vi "Begin.vi"(8 "error in":errorcluster) -> (0 "error out":errorcluster)   [LabVIEW 2016]
doc: "Called before other user functions, this VI is expected to open initial I/O refnums, load in file data, and do all program initialization. Notice that the <B>error out</B> terminal is simply used for data flow. Wiring it to other structures or subVIs ensures that this VI runs first."
uses:
  <vilib>/Rock Robotics/WPI/SafetyOutput/WPI_SafetyOutputConfigMenu.ctl
  <vilib>/Rock Robotics/WPI/DriverStation/WPI_DriverStationRobotMode2.ctl
  <vilib>/Rock Robotics/WPI/Joystick/WPI_JoystickDeviceEnum.ctl
  <vilib>/Rock Robotics/SystemInterfaces/DIO/FPGA_DIOPWMChannel.ctl
  <vilib>/Rock Robotics/WPI/ThirdParty/CanMotor/TalonSRX/WPI_CANTalonSRX_APIControlMode.ctl
  <vilib>/Rock Robotics/WPI/ThirdParty/CanMotor/TalonSRX/WPI_CANTalonSRX_APIFeedbackSelect.ctl
  navx-mxp/labview/NI WPI/WPI_SerialPort_USB.ctl
  navx-mxp/labview/navX Library v2/TypeDefs/Z900_navX_SerialStreamTypeDef.ctl
  <vilib>/Rock Robotics/SystemInterfaces/DIO/FPGA_DIORelayChannel.ctl
  <vilib>/Rock Robotics/SystemInterfaces/DIO/FPGA_DIOChannel.ctl
  <vilib>/Rock Robotics/WPI/Relay/WPI_RelayValue.ctl
  <vilib>/Rock Robotics/WPI/ThirdParty/CanMotor/TalonSRX/WPI_CANTalonSRX_BrakeOverride.ctl
  Robot Global Data.vi
  <vilib>/Rock Robotics/Network Tables/NT Write String Array.vi
  <vilib>/Rock Robotics/WPI/MotorControl/WPI_MotorControlOpen Victor.vi
  navx-mxp/labview/navX Library v2/IO/Open/Z900_navX_Open_Serial.vi
  <vilib>/Rock Robotics/WPI/Switch/WPI_SwitchOpenLimit.vi
  navx-mxp/labview/navX Library v2/navX Library v2.lvlib
  navx-mxp/labview/NI WPI/NI WPI Serial USB.lvlib
  <vilib>/Rock Robotics/SystemInterfaces/i2clib/i2c_bus.ctl
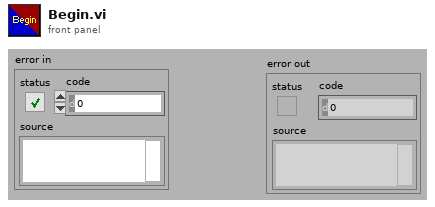
[diagram p1: front panel]
types:
  T1 = typedef "WPI_CANTalonSRX_BrakeOverride.ctl" = enum8{"No Override", "Override to Coast", "Override to Brake"}
  T2 = typedef "WPI_RelayValue.ctl" = enum16{"Off", "On", "Forward", "Reverse"}
  T3 = typedef "FPGA_DIORelayChannel.ctl" = enum8{"Relay 0", "Relay 1", "Relay 2", "Relay 3", "Invalid"}
  T4 = typedef "WPI_JoystickDeviceEnum.ctl" = enum16{"USB 0", "USB 1", "USB 2", "USB 3", "USB 4", "USB 5"}
  T5 = typedef "FPGA_DIOChannel.ctl" = enum8{"DIO 0", "DIO 1", "DIO 2", "DIO 3", "DIO 4", "DIO 5", "DIO 6", "DIO 7", "DIO 8", "DIO 9", "DIO MXP 0", "DIO MXP 1", "DIO MXP 2", "DIO MXP 3", "DIO MXP 4", "DIO MXP 5", "DIO MXP 6", "DIO MXP 7", "DIO MXP 8", "DIO MXP 9", "DIO MXP 10", "DIO MXP 11", "DIO MXP 12", "DIO MXP 13", "DIO MXP 14", "DIO MXP 15", "SPI Port CS1", "SPI Port CS2", "SPI Port CS3", "SPI Port MISO", "SPI Port MOSI", "Invalid"}
  T6 = typedef "WPI_CANTalonSRX_APIFeedbackSelect.ctl" = enum16{"Digital Quadrature Encoder", "Analog Potentiometer", "Analog Encoder", "Count on Quad-A (Rising-Edge)", "Count on Quad-A (Falling-Edge)", "CTR Magnetic Enc (Absolute)", "CTR Magnetic Enc (Relative)", "Pulse Width"}
  T7 = typedef "WPI_CANTalonSRX_APIControlMode.ctl" = enum8{"Percent VBus", "Speed", "Position", "Slave", "Unchanged / Invalid", "Voltage Compensation", "Current", "Motion Profile", "Motion Magic"}
  T8 = typedef "FPGA_DIOPWMChannel.ctl" = enum8{"PWM 0", "PWM 1", "PWM 2", "PWM 3", "PWM 4", "PWM 5", "PWM 6", "PWM 7", "PWM 8", "PWM 9", "PWM MXP 0", "PWM MXP 1", "PWM MXP 2", "PWM MXP 3", "PWM MXP 4", "PWM MXP 5", "PWM MXP 6", "PWM MXP 7", "PWM MXP 8", "PWM MXP 9", "Invalid"}
  T9 = typedef "navX Library v2.lvlib/Z900_navX_SerialStreamTypeDef.ctl" = enum16{"YRPH", "Quaterinons", "Gyro/Raw", "AHRS", "AHRSAndPositioning"}
  T10 = typedef "NI WPI Serial USB.lvlib/WPI_SerialPort_USB.ctl" = enum16{"Onboard RS-232", "MXP TTL", "USB"}
  T11 = typedef "WPI_DriverStationRobotMode2.ctl" = enum16{"Autonomous Disabled", "Autonomous Enabled", "Teleop Disabled", "Teleop Enabled", "Disconnected", "Finish", "Test Disabled", "Test Enabled", "Emergency Stopped"}
  T12 = typedef "WPI_SafetyOutputConfigMenu.ctl" = enum16{"Enable", "Disable"}
  T13 = typedef "i2c_bus.ctl" = enum16{"I2C On-Board", "I2C MXP", "Invalid"}
  T14 = typedef "WPI_I2CDevRef.ctl" = cluster{"DevStatus":errorcluster, "Device Address":u8, "Handle":i32, "I2C Bus":T13}
  T15 = typedef "WPI_JoystickDevRef.ctl" = cluster{"Device":T4}
  T16 = typedef "WPI_RobotDriveDevRef.ctl" = cluster{"DevStatus":errorcluster, "Motors[]":T17[], "Square Inputs":bool, "Max Output":dbl}
  T17 = typedef "WPI_MotorControlDeviceRef.ctl" = cluster{"DeviceStatus":errorcluster, "Type":T18, "PWM":cluster{"PWM Channel":T8, "DeadBand":T19}, "CAN":cluster{"Device Number":u8, "SetOutput VI Ref":variant, "GetOutput VI Ref":variant, "Enable VI Ref":variant, "Disable VI Ref":variant, "Data":variant}, "Invert":bool}
  T18 = typedef "WPI_MotorControlType.ctl" = enum16{"PWM", "CAN"}
  T19 = typedef "WPI_PWMDeadband.ctl" = cluster{"Name":string, "maxPositivePwm":i32, "minPositivePwm":i32, "centerPwm":i32, "maxNegativePwm":i32, "minNegativePwm":i32, "angularRange":u16}
  T20 = typedef "navX Library v2.lvlib/Z900_navX_DeviceTypeDef.ctl" = cluster{"Interface":cluster{"Protocol":T21, "Update Rate (4Hz-100Hz)":u8, "navX Open TypeDef":variant}, "Notify Packet":refnum<notifier>, "Loop VI Refnum":refnum<vi>, "Ready to Close Occurrence Refnum":refnum<k4>}
  T21 = typedef "navX Library v2.lvlib/Z900_navX_ProtocolTypeDef.ctl" = enum16{"SERIAL", "I2C", "SPI"}
  T22 = typedef "WPI_SwitchDevRef.ctl" = cluster{"DevStatus":errorcluster, "DIO Channel":T5, "CntIndex":T23, "Normally Closed":bool}
  T23 = typedef "FPGA_CounterCtrSystemIndex.ctl" = enum8{"Ctr 0", "Ctr 1", "Ctr 2", "Ctr 3", "Ctr 4", "Ctr 5", "Ctr 6", "Ctr 7", "Invalid"}
  T24 = typedef "WPI_RelayDevRef.ctl" = cluster{"DevStatus":errorcluster, "Relay Channel":T3, "Relay Direction":T25}
  T25 = typedef "WPI_RelayDirection.ctl" = enum16{"Both directions", "Forward only", "Reverse only"}
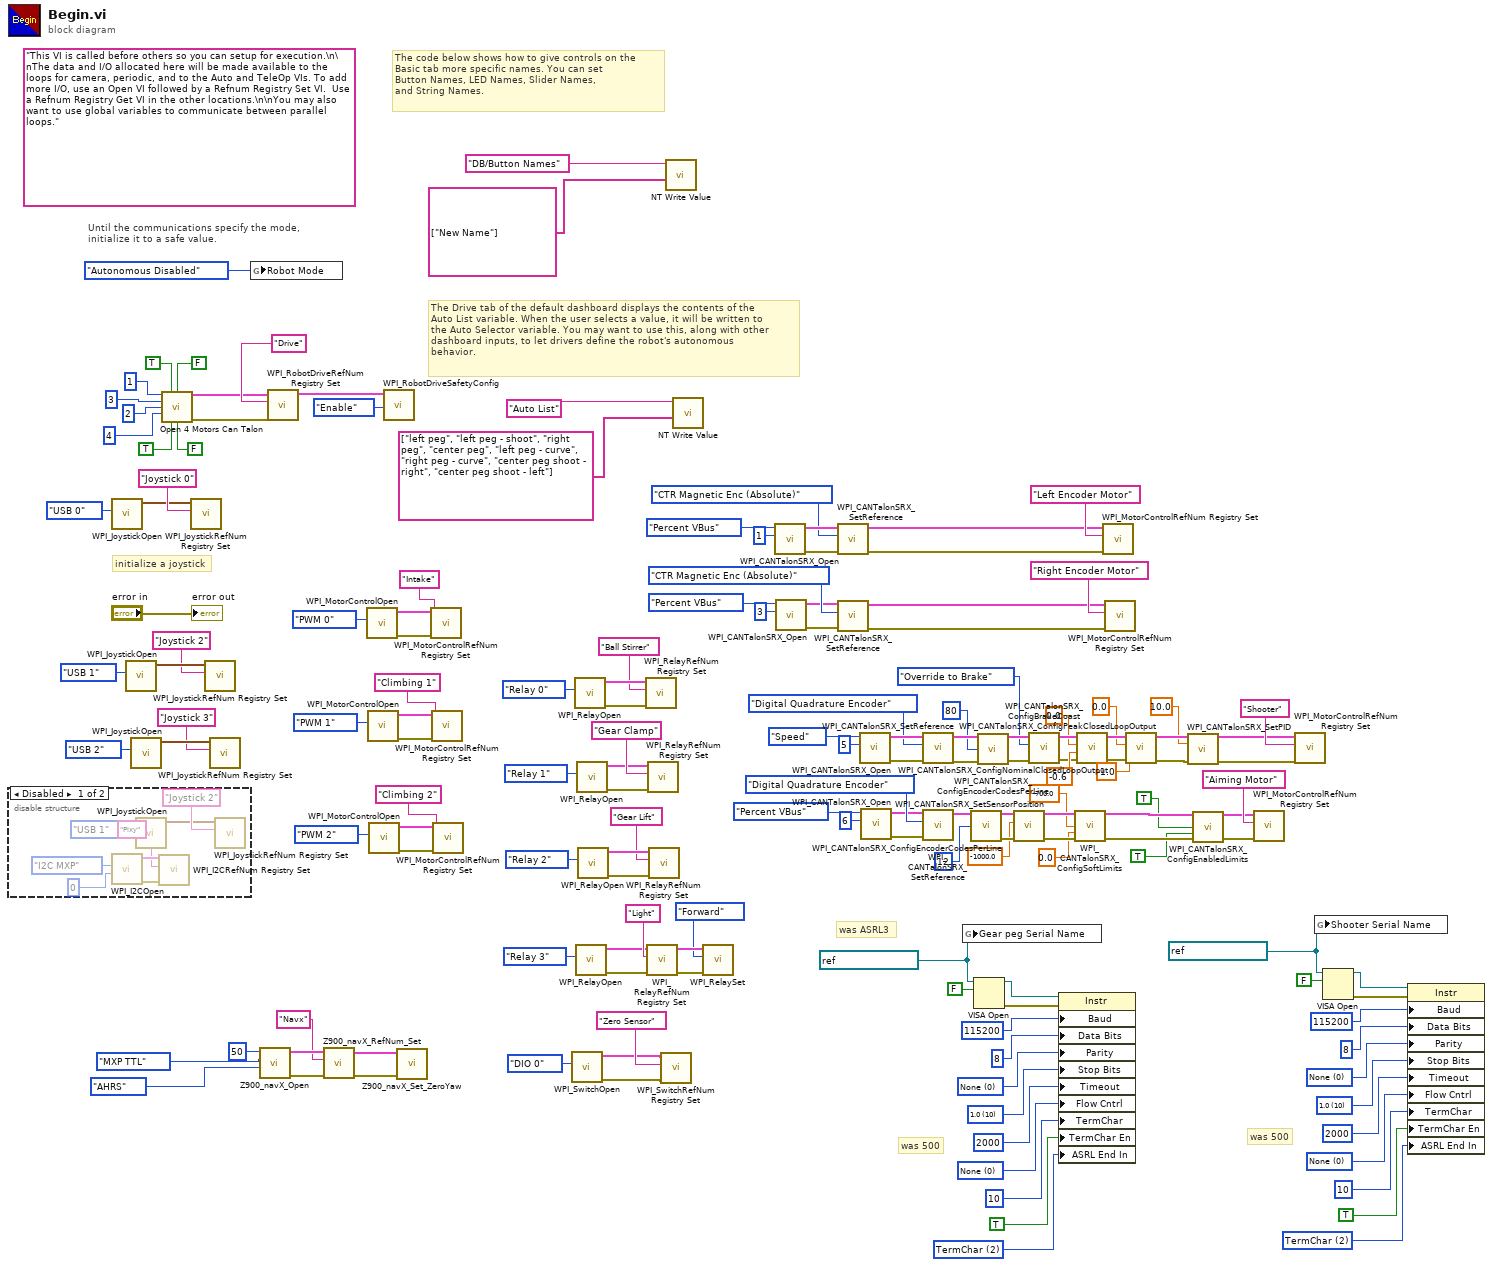
[diagram p0: block diagram]
diagram:
  w30 = refnum<visa-resource-name> "ASRL3::INSTR" ("VISA Refnum out")
  w29 = u16 2 items=["None", "Last Bit", "TermChar"] ("Serial Settings:End Mode for Reads")
  w26 = u16 0 items=["None", "XON/XOFF", "RTS/CTS", "XON/XOFF & RTS/CTS", "DTR/DSR", "XON/XOFF & DTR/DSR"] ("Flow Control")
  w24 = u16 10 items=["1.0"=10, "1.5"=15, "2.0"=20] ("Stop Bits")
  w23 = u16 0 items=["None", "Odd", "Even", "Mark", "Space"] ("Parity")
  w102 = refnum<visa-resource-name> "ASRL4::INSTR" ("VISA Refnum out")
  w103 = u16 2 items=["None", "Last Bit", "TermChar"] ("Serial Settings:End Mode for Reads")
  w106 = u16 0 items=["None", "XON/XOFF", "RTS/CTS", "XON/XOFF & RTS/CTS", "DTR/DSR", "XON/XOFF & DTR/DSR"] ("Flow Control")
  w108 = u16 10 items=["1.0"=10, "1.5"=15, "2.0"=20] ("Stop Bits")
  w109 = u16 0 items=["None", "Odd", "Even", "Mark", "Space"] ("Parity")
  (unwired) "This VI is called before others so you can setup for execution.\n\nThe data and I/O allocated here will be made available to the loops for camera, periodic, and to the Auto and TeleOp VIs. To add more I/O, use an Open VI followed by a Refnum Registry Set VI.  Use a Refnum Registry Get VI in the other locations.\n\nYou may also want to use global variables to communicate between parallel loops."
  # "was ASRL3"
  # "was 500"
  # "was 500"
  # "The Drive tab of the default dashboard displays the contents of the\nAuto List variable. When the user selects a value, it will be written to\nthe Auto Selector variable. You may want to use this, along with other\ndashboard inputs, to let drivers define the robot's autonomous\nbehavior."
  # "The code below shows how to give controls on the\nBasic tab more specific names. You can set\nButton Names, LED Names, Slider Names,\nand String Names."
  # "initialize a joystick"
  # "Until the communications specify the mode,\ninitialize it to a safe value."
  n1 = disable-structure shown="Disabled" {
    frame Disabled {
      n2 = call <vilib>:"WPI_I2COpen.vi"("Device Address"=u8 0, "I2C Bus"=i2c_bus."I2C MXP") -> ("error out"=w162:errorcluster, "I2CDevRef"=w161:T14)  [unwired: 8 in]
      n3 = call <vilib>:"WPI_JoystickOpen.vi"("JoystickDevice"=WPI_JoystickDeviceEnum."USB 1") -> ("JoystickDevRef"=w158:T15)  [unwired: 10 in]
      n4 = call <vilib>:"WPI_I2CRefNum Registry Set.vi"("error in (no error)"=w162, "refnum name"="Pixy", "I2CDevRef"=w161) -> ()  [unwired: 7 in, 2 out]
      n5 = call <vilib>:"WPI_JoystickRefNum Registry Set.vi"("refnum name"="Joystick 2", "JoystickDevRef"=w158) -> ()  [unwired: 8 in, 2 out]
    }
    frame Enabled {
    }
  }
  n6 = call <vilib>:"WPI_JoystickOpen.vi"("JoystickDevice"=WPI_JoystickDeviceEnum."USB 0") -> ("JoystickDevRef"=w151:T15)  [unwired: 10 in]
  n7 = call <vilib>:"WPI_JoystickOpen.vi"("JoystickDevice"=WPI_JoystickDeviceEnum."USB 1") -> ("JoystickDevRef"=w65:T15)  [unwired: 10 in]
  n8 = call <vilib>:"WPI_JoystickOpen.vi"("JoystickDevice"=WPI_JoystickDeviceEnum."USB 2") -> ("JoystickDevRef"=w51:T15)  [unwired: 10 in]
  n9 = call <vilib>:"Open 4 Motors Can Talon.vi"("Rear Left Motor"=u8 1, "Rear Left Motor Inverted"=TRUE, "Rear Right Motor Inverted"=FALSE, "Rear Right Motor"=u8 3, "Front Left Motor"=u8 2, "Front Right Motor"=u8 4, "Front Left Motor Inverted"=TRUE, "Front Right Motor Inverted"=FALSE) -> ("RobotDriveDevRef"=w140:T16, "error out"=w139:errorcluster)  [unwired: 6 in]
  n10 = call <vilib>:"WPI_JoystickRefNum Registry Set.vi"("refnum name"="Joystick 0", "JoystickDevRef"=w151) -> ()  [unwired: 8 in, 2 out]
  n11 = call <vilib>:"WPI_JoystickRefNum Registry Set.vi"("refnum name"="Joystick 2", "JoystickDevRef"=w65) -> ()  [unwired: 8 in, 2 out]
  n12 = call <vilib>:"WPI_JoystickRefNum Registry Set.vi"("refnum name"="Joystick 3", "JoystickDevRef"=w51) -> ()  [unwired: 8 in, 2 out]
  n13 = global write "Robot Global Data.vi" "Robot Mode"(WPI_DriverStationRobotMode2."Autonomous Disabled" ("Robot Mode")) -> ()
  n14 = call-poly "Z900_navX_Open.vi"("Stream Type"=Z900_navX_SerialStreamTypeDef."AHRS", "Serial Port"=WPI_SerialPort_USB."MXP TTL", "Update Rate (4Hz-60Hz)"=u8 50) -> ("error out"=w119:errorcluster, "navX Device"=w120:T20)  [unwired: 7 in]
  n15 = call <vilib>:"WPI_RobotDriveRefNum Registry Set.vi"("error in (no error)"=w139, "refnum name"="Drive", "RobotDriveDevRef"=w140) -> ("RobotDriveDevRef"=w155:T16)  [unwired: 1 in, 7 out]
  n16 = call "Z900_navX_RefNum_Set.vi"("error in (no error)"=w119, "refnum name"="Navx", "navX Device"=w120) -> ("error out"=w94:errorcluster, "navX Device"=w95:T20)  [unwired: 7 in]
  n17 = call-poly <vilib>:"WPI_MotorControlOpen.vi"("PWM Channel"=FPGA_DIOPWMChannel."PWM 0") -> ("error out"=w132:errorcluster, "MotorControlDeviceRef"=w133:T17)  [unwired: 9 in]
  n18 = call-poly <vilib>:"WPI_MotorControlOpen.vi"("PWM Channel"=FPGA_DIOPWMChannel."PWM 1") -> ("error out"=w92:errorcluster, "MotorControlDeviceRef"=w91:T17)  [unwired: 9 in]
  n19 = call-poly <vilib>:"WPI_MotorControlOpen.vi"("PWM Channel"=FPGA_DIOPWMChannel."PWM 2") -> ("error out"=w87:errorcluster, "MotorControlDeviceRef"=w88:T17)  [unwired: 9 in]
  n20 = call <vilib>:"WPI_RobotDriveSafetyConfig.vi"("mode"=WPI_SafetyOutputConfigMenu."Enable", "RobotDriveDevRef"=w155) -> ()  [unwired: 8 in, 2 out]
  n21 = call "Z900_navX_Set_ZeroYaw.vi"("error in (no error)"=w94, "navX Device"=w95) -> ()  [unwired: 8 in, 2 out]
  n22 = call <vilib>:"WPI_MotorControlRefNum Registry Set.vi"("error in (no error)"=w132, "refnum name"="Intake", "MotorControlDevRef"=w133) -> ()  [unwired: 7 in, 2 out]
  n23 = call <vilib>:"WPI_MotorControlRefNum Registry Set.vi"("error in (no error)"=w92, "refnum name"="Climbing 1", "MotorControlDevRef"=w91) -> ()  [unwired: 7 in, 2 out]
  n24 = call <vilib>:"WPI_MotorControlRefNum Registry Set.vi"("error in (no error)"=w87, "refnum name"="Climbing 2", "MotorControlDevRef"=w88) -> ()  [unwired: 7 in, 2 out]
  n25 = call-poly <vilib>:"WPI_SwitchOpen.vi"("DIO Channel"=FPGA_DIOChannel."DIO 0") -> ("error out"=w53:errorcluster, "SwitchDevRef"=w54:T22)  [unwired: 9 in]
  n26 = call <vilib>:"WPI_RelayOpen.vi"("Relay Channel"=FPGA_DIORelayChannel."Relay 0") -> ("error out"=w85:errorcluster, "RelayDevRef"=w84:T24)  [unwired: 9 in]
  n27 = call <vilib>:"WPI_RelayOpen.vi"("Relay Channel"=FPGA_DIORelayChannel."Relay 3") -> ("error out"=w46:errorcluster, "RelayDevRef"=w47:T24)  [unwired: 9 in]
  n28 = call <vilib>:"WPI_RelayOpen.vi"("Relay Channel"=FPGA_DIORelayChannel."Relay 1") -> ("error out"=w60:errorcluster, "RelayDevRef"=w61:T24)  [unwired: 9 in]
  n29 = call <vilib>:"WPI_RelayOpen.vi"("Relay Channel"=FPGA_DIORelayChannel."Relay 2") -> ("error out"=w59:errorcluster, "RelayDevRef"=w58:T24)  [unwired: 9 in]
  n30 = call <vilib>:"WPI_RelayRefNum Registry Set.vi"("error in (no error)"=w85, "refnum name"="Ball Stirrer", "RelayDevRef"=w84) -> ()  [unwired: 7 in, 2 out]
  n31 = call <vilib>:"WPI_RelayRefNum Registry Set.vi"("error in (no error)"=w46, "refnum name"="Light", "RelayDevRef"=w47) -> ("error out"=w45:errorcluster, "RelayDevRef"=w44:T24)  [unwired: 7 in]
  n32 = call <vilib>:"WPI_RelayRefNum Registry Set.vi"("error in (no error)"=w60, "refnum name"="Gear Clamp", "RelayDevRef"=w61) -> ()  [unwired: 7 in, 2 out]
  n33 = call <vilib>:"WPI_RelayRefNum Registry Set.vi"("error in (no error)"=w59, "refnum name"="Gear Lift", "RelayDevRef"=w58) -> ()  [unwired: 7 in, 2 out]
  n34 = call <vilib>:"WPI_SwitchRefNum Registry Set.vi"("error in (no error)"=w53, "refnum name"="Zero Sensor", "SwitchDevRef"=w54) -> ()  [unwired: 7 in, 2 out]
  n35 = call-poly <vilib>:"NT Write Value.vi"("String Array"=string[] ["New Name"], "Name"="DB/Button Names") -> ()  [unwired: 9 in, 1 out]
  n36 = call-poly <vilib>:"NT Write Value.vi"("String Array"=string[] ["left peg", "left peg - shoot", "right peg", "center peg", "left peg - curve", "right peg - curve", "center peg shoot - right", "center peg shoot - left"], "Name"="Auto List") -> ()  [unwired: 9 in, 1 out]
  n37 = call <vilib>:"WPI_RelaySet.vi"("error in (no error)"=w45, "RelayValue"=WPI_RelayValue."Forward", "RelayDevRef"=w44) -> ()  [unwired: 7 in, 2 out]
  n38 = call <vilib>:"WPI_CANTalonSRX_Open.vi"("Device Number"=u8 1, "Control Mode"=WPI_CANTalonSRX_APIControlMode."Percent VBus") -> ("error out"=w125:errorcluster, "CAN Talon SRX Ref"=w126:T17)  [unwired: 8 in]
  n39 = call <vilib>:"WPI_CANTalonSRX_Open.vi"("Device Number"=u8 3, "Control Mode"=WPI_CANTalonSRX_APIControlMode."Percent VBus") -> ("error out"=w100:errorcluster, "CAN Talon SRX Ref"=w101:T17)  [unwired: 8 in]
  n40 = call <vilib>:"WPI_CANTalonSRX_SetReference.vi"("error in (no error)"=w125, "Feedback Reference"=WPI_CANTalonSRX_APIFeedbackSelect."CTR Magnetic Enc (Absolute)", "CAN Talon SRX Ref"=w126) -> ("error out"=w96:errorcluster, "CAN Talon SRX Ref"=w97:T17)  [unwired: 7 in]
  n41 = call <vilib>:"WPI_CANTalonSRX_SetReference.vi"("error in (no error)"=w100, "Feedback Reference"=WPI_CANTalonSRX_APIFeedbackSelect."CTR Magnetic Enc (Absolute)", "CAN Talon SRX Ref"=w101) -> ("error out"=w98:errorcluster, "CAN Talon SRX Ref"=w99:T17)  [unwired: 7 in]
  n42 = call <vilib>:"WPI_CANTalonSRX_Open.vi"("Device Number"=u8 5, "Control Mode"=WPI_CANTalonSRX_APIControlMode."Speed") -> ("error out"=w76:errorcluster, "CAN Talon SRX Ref"=w77:T17)  [unwired: 8 in]
  n43 = call <vilib>:"WPI_CANTalonSRX_Open.vi"("Device Number"=u8 6, "Control Mode"=WPI_CANTalonSRX_APIControlMode."Percent VBus") -> ("error out"=w70:errorcluster, "CAN Talon SRX Ref"=w71:T17)  [unwired: 8 in]
  n44 = call <vilib>:"WPI_CANTalonSRX_SetReference.vi"("error in (no error)"=w76, "Feedback Reference"=WPI_CANTalonSRX_APIFeedbackSelect."Digital Quadrature Encoder", "CAN Talon SRX Ref"=w77) -> ("error out"=w15:errorcluster, "CAN Talon SRX Ref"=w68:T17)  [unwired: 7 in]
  n45 = call <vilib>:"WPI_CANTalonSRX_SetReference.vi"("error in (no error)"=w70, "Feedback Reference"=WPI_CANTalonSRX_APIFeedbackSelect."Digital Quadrature Encoder", "CAN Talon SRX Ref"=w71) -> ("CAN Talon SRX Ref"=w69:T17)  [unwired: 7 in, 1 out]
  n46 = global write "Robot Global Data.vi" "Gear peg Serial Name"(w102) -> ()
  n47 = call <vilib>:"WPI_CANTalonSRX_ConfigEncoderCodesPerLine.vi"("CAN Talon SRX Ref"=w69, "Number Encoder Lines\n(Counts Per Rotation)"=u32 12 ("Number Encoder Lines\n(Counts Per Rotation)")) -> ("CAN Talon SRX Ref"=w40:T17, "error out"=w41:errorcluster)  [unwired: 12 in]
  n48 = VISA Open(duplicate session (F)=FALSE, VISA resource name=w102) -> (VISA resource name=w114:refnum<visa-resource-name>, error out=w113:errorcluster)  [unwired: 1 in, 2 out]
  n49 = call <vilib>:"WPI_CANTalonSRX_ConfigEncoderCodesPerLine.vi"("CAN Talon SRX Ref"=w68, "Number Encoder Lines\n(Counts Per Rotation)"=u32 80 ("Number Encoder Lines\n(Counts Per Rotation)"), "error in (no error)"=w15) -> ("CAN Talon SRX Ref"=w17:T17, "error out"=w13:errorcluster)  [unwired: 11 in]
  n50 = call <vilib>:"WPI_CANTalonSRX_SetSensorPosition.vi"("error in (no error)"=w41, "New Sensor Position"=-1000.0, "CAN Talon SRX Ref"=w40) -> ("error out"=w38:errorcluster, "CAN Talon SRX Ref"=w39:T17)  [unwired: 7 in]
  n51 = call <vilib>:"WPI_CANTalonSRX_ConfigBrakeCoast.vi"("error in (no error)"=w13, "Brake / Coast Mode"=WPI_CANTalonSRX_BrakeOverride."Override to Brake", "CAN Talon SRX Ref"=w17) -> ("error out"=w6:errorcluster, "CAN Talon SRX Ref"=w14:T17)  [unwired: 7 in]
  n52 = property class="Instr"(reference=w114, error in=w113, "Baud"=u32 115200 ("Baud Rate"), "Data Bits"=u16 8, "Parity"=w109, "Stop Bits"=w108, "Timeout"=u32 2000 ("Timeout Value (ms)"), "Flow Cntrl"=w106, "TermChar"=u8 10 ("Termination Char (0xA = '\\n' = LF)"), "TermChar En"=TRUE ("Message Based Settings:Termination Character Enable"), "ASRL End In"=w103) -> ()  [unwired: 2 out]
  n53 = call <vilib>:"WPI_CANTalonSRX_ConfigSoftLimits.vi"("CAN Talon SRX Ref"=w39, "Forward Limit Position"=-700.0 ("Reverse Limit Position"), "Reverse Limit Position"=0.0 ("Forward Limit Position")) -> ("CAN Talon SRX Ref"=w36:T17)  [unwired: 11 in, 1 out]
  n54 = call <vilib>:"WPI_CANTalonSRX_ConfigNominalClosedLoopOutput.vi"("Reverse Nominal Output"=-0.6, "Forward Nominal Output"=0.0, "CAN Talon SRX Ref"=w14) -> ("CAN Talon SRX Ref"=w11:T17)  [unwired: 7 in, 1 out]
  n55 = call <vilib>:"WPI_MotorControlRefNum Registry Set.vi"("error in (no error)"=w96, "refnum name"="Left Encoder Motor", "MotorControlDevRef"=w97) -> ()  [unwired: 7 in, 2 out]
  n56 = call <vilib>:"WPI_MotorControlRefNum Registry Set.vi"("error in (no error)"=w98, "refnum name"="Right Encoder Motor", "MotorControlDevRef"=w99) -> ()  [unwired: 7 in, 2 out]
  n57 = call <vilib>:"WPI_CANTalonSRX_ConfigPeakClosedLoopOutput.vi"("error in (no error)"=w6, "Reverse Peak Output"=-1.0, "Forward Peak Output"=0.0, "CAN Talon SRX Ref"=w11) -> ("error out"=w2:errorcluster, "CAN Talon SRX Ref"=w9:T17)  [unwired: 6 in]
  n58 = call <vilib>:"WPI_CANTalonSRX_SetPID.vi"("CAN Talon SRX Ref"=w9, "P"=10.0, "error in (no error)"=w2) -> ("CAN Talon SRX Ref"=w4:T17, "error out"=w1:errorcluster)  [unwired: 11 in]
  n59 = call <vilib>:"WPI_CANTalonSRX_ConfigEnabledLimits.vi"("CAN Talon SRX Ref"=w36, "Forward Limit Switch Enable"=TRUE, "Reverse Limit Switch Enable"=TRUE) -> ("CAN Talon SRX Ref"=w35:T17)  [unwired: 11 in, 1 out]
  n60 = call <vilib>:"WPI_MotorControlRefNum Registry Set.vi"("error in (no error)"=w38, "refnum name"="Aiming Motor", "MotorControlDevRef"=w35) -> ()  [unwired: 7 in, 2 out]
  n61 = call <vilib>:"WPI_MotorControlRefNum Registry Set.vi"("error in (no error)"=w1, "refnum name"="Shooter", "MotorControlDevRef"=w4) -> ()  [unwired: 7 in, 2 out]
  n62 = global write "Robot Global Data.vi" "Shooter Serial Name"(w30) -> ()
  n63 = VISA Open(duplicate session (F)=FALSE, VISA resource name=w30) -> (VISA resource name=w18:refnum<visa-resource-name>, error out=w19:errorcluster)  [unwired: 1 in, 2 out]
  n64 = property class="Instr"(reference=w18, error in=w19, "Baud"=u32 115200 ("Baud Rate"), "Data Bits"=u16 8, "Parity"=w23, "Stop Bits"=w24, "Timeout"=u32 2000 ("Timeout Value (ms)"), "Flow Cntrl"=w26, "TermChar"=u8 10 ("Termination Char (0xA = '\\n' = LF)"), "TermChar En"=TRUE ("Message Based Settings:Termination Character Enable"), "ASRL End In"=w29) -> ()  [unwired: 2 out]
  "error out" <- "error in"
